vi "Name Prompt UI.vi"(11 "Initial Name (Empty)":string) -> (2 "Cancelled":bool, 3 "Name":string)   [LabVIEW 2020, in "Negentropic IDE.lvlib"]
uses:
  Negentropic IDE.lvlib
panel:
  in  "Cancel":bool
  in  "OK":bool
  in  "Name Entry":string
  # "Enter name for folder layout , this will be the name that shows up in the menu:"
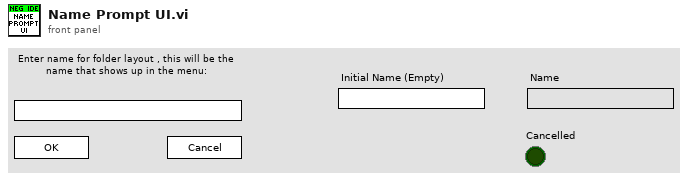
[diagram p1: front panel]
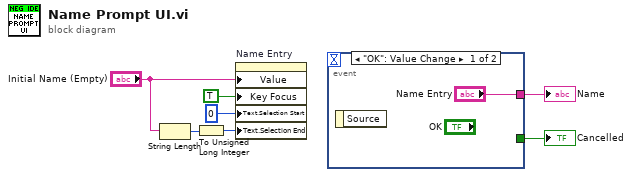
[diagram p0: block diagram]
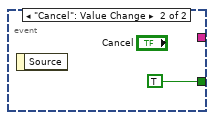
[diagram p2: hidden frame]
diagram:
  n1 = String Length(string="Initial Name (Empty)") -> (length=w4:i32)
  n2 = To Unsigned Long Integer(number=w4) -> (unsigned 32bit integer=w2:u32)
  n3 = property on="Name Entry" class="Str"("Value"="Initial Name (Empty)", "Key Focus"=TRUE, "Text.Selection Start"=u32 0 ("Text.Selection:Start"), "Text.Selection End"=w2) -> ()  [unwired: 2 in, 2 out]
  n4 = event shown="[0] \"OK\": Value Change" {
    selector: _ -> [_ _]
    dyn-events: _ -> [_ _]
    timeout: _ -> [_ _]
    tunnel: ["Name Entry" _] -> w6
    tunnel: [_ TRUE] -> w5
    event "OK": Value Change {
      n5 = event-data() -> ()  [unwired: 1 in, 1 out]
    }
    event "Cancel": Value Change {
      n6 = event-data() -> ()  [unwired: 1 in, 1 out]
    }
  }
  "Name" <- w6
  "Cancelled" <- w5
